vi "Get Folder Tag.vi"(7 "Selected cell Tag":string) -> (3 "Folder Tag":string)   [LabVIEW 2021, in "Converter.lvlib"]
uses:
  Converter.lvlib
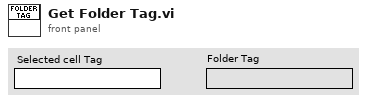
[diagram p1: front panel]
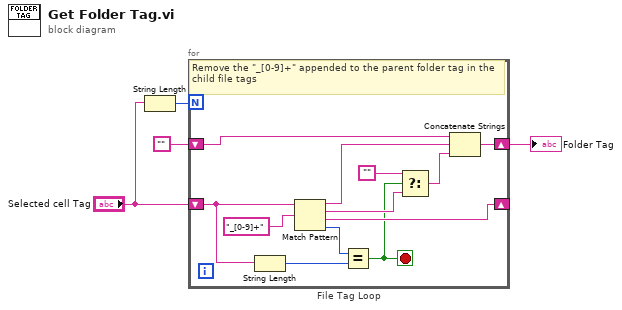
[diagram p0: block diagram]
diagram:
  n1 = String Length(string="Selected cell Tag") -> (length=w4:i32)
  n2 = for "File Tag Loop" {
    N: w4 -> [_]
    shift-right: [w12] -> _
    shift-left: "Selected cell Tag" -> [w15]
    shift-right: [w9] -> w1
    shift-left: "" -> [w8]
    stop <- w10 stop-if-true
    # "Remove the \"_[0-9]+\" appended to the parent folder tag in the child file tags"
    n3 = String Length(string=w15) -> (length=w14:i32)
    n4 = Match Pattern(string=w15, regular expression="_[0-9]+") -> (before substring=w6:string, match substring=w11:string, after substring=w12:string, offset past match=w13:i32)  [unwired: 1 in]
    n5 = Equal?(x=w13, y=w14) -> (x = y?=w10:bool)
    n6 = Select(t="", s=w10, f=w11) -> (s? t:f=w7:string)
    n7 = Concatenate Strings(w8, w6, w7) -> (w9:string)
  }
  "Folder Tag" <- w1
